vi "Set Speed.vi"(6 "Units (0: data)":u16(ring) items=["device units", "microns/s", "mm/s", "inches/s", "degrees/s"], 7 "New Speed":dbl, 8 "error in (no error)":errorcluster, 9 "Device and Axis":string, 10 "Microstep Size (0)":dbl, 11 "VISA resource name":refnum<visa-resource-name>) -> (0 "error out":errorcluster, 3 "VISA resource name out":refnum<visa-resource-name>)   [LabVIEW 2015, in "Zaber A Series.lvlib"]
doc: "Sets the maximum speed of a device to a new value. The desired speed and units of measure are inputs. If the speed input is zero, then it won't be updated. The units for the maximum speed can be selected with the Units input. 'Data' units are the default, and other unit selections require the Microstep Size for the device to be input. If you'd like to specify a Device and Axis to adjust the settings of, specify this input.\n\nThis VI requires that the Initialize VI has been called with the same serial port."
uses:
  Zaber A Series.lvlib
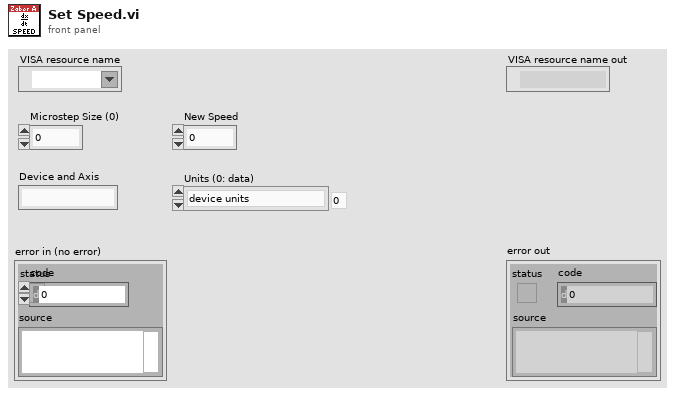
[diagram p1: front panel]
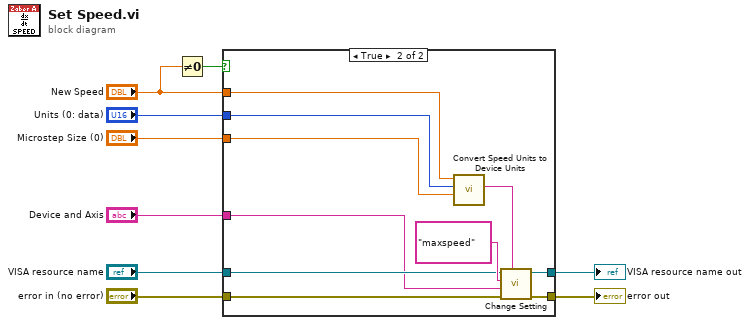
[diagram p0: block diagram]
diagram:
  n1 = Not Equal To 0?(x="New Speed") -> (x != 0?=w6:bool)
  n2 = case shown="True" w6 {
    tunnel: "VISA resource name" -> [w11 w19]
    tunnel: "error in (no error)" -> [w10 w20]
    tunnel: "New Speed" -> [_ w12]
    tunnel: "Microstep Size (0)" -> [_ w14]
    tunnel: "Units (0: data)" -> [_ w13]
    tunnel: [w11 w18] -> w2
    tunnel: [w10 w17] -> w1
    tunnel: "Device and Axis" -> [_ w15]
    frame False {
    }
    frame True {
      n3 = call "Convert Speed Units to Device Units.vi"("Microstep Size (0)"=w14, "Units (0: device speed units)"=w13, "Speed (0)"=w12) -> ("Device Speed (String)"=w16:string)  [unwired: 6 in, 2 out]
      n4 = call "Change Setting.vi"("Data"=w16, "error in (no error)"=w20, "Device and Axis"=w15, "Setting"="maxspeed" ("Common Settings"), "VISA resource name"=w19) -> ("error out"=w17:errorcluster, "VISA resource name out"=w18:refnum<visa-resource-name>)  [unwired: 5 in]
    }
  }
  "VISA resource name out" <- w2
  "error out" <- w1
